vi "LVFunction_Imop_Compute_ModalWavefront.vi"(0 "HasoData":refnum<class "HasoData.lvclass">, 5 "ComputePhaseSet":refnum<class "ComputePhaseSet.lvclass">, 7 "Phase":refnum<class "Phase.lvclass">, 9 "ModalCoef.lvclass":refnum<class "ModalCoef.lvclass">, 11 "error constant":errorcluster) -> (4 "HasoData (dup)":refnum<class "HasoData.lvclass">, 6 "ComputePhaseSet (dup)":refnum<class "ComputePhaseSet.lvclass">, 8 "Phase.lvclass":refnum<class "Phase.lvclass">, 10 "ModalCoef.lvclass (dup)":refnum<class "ModalCoef.lvclass">, 15 "error out":errorcluster)   [LabVIEW 2018]
doc: "Compute phase from processed slopes of the input HasoData via modal\ncoefficients in a given basis of polynomials provided by ComputePhaseSet.\n\n<B>ComputePhaseSetIn</B> : ComputePhaseSet object.\n<B>ComputePhaseSetOut</B> : ComputePhaseSet object.\n<B>HasoData</B> : HasoData object.\n<B>ModalCoeffs</B> : ModalCoef object. Preferences are used as input, coefficients values are updated by the processing.\n<B>Phase</B> : phase object. Phase values and steps are expressed in um."
uses:
  Classes/HasoData/HasoData.lvclass
  Classes/ComputePhaseSet/ComputePhaseSet.lvclass
  Classes/Phase/Phase.lvclass
  Classes/ModalCoef/ModalCoef.lvclass
  Classes/ModalCoef/LVClass_ModalCoef Read ModalCoef.vi
  Classes/Phase/LVClasse_Phase Read SurfaceFloatWithPupil.vi
  Classes/ComputePhaseSet/LVClass_ComputePhaseSet Read ComputePhaseSet.vi
  Classes/HasoData/LVClass_HasoData Read HasoData - property.vi
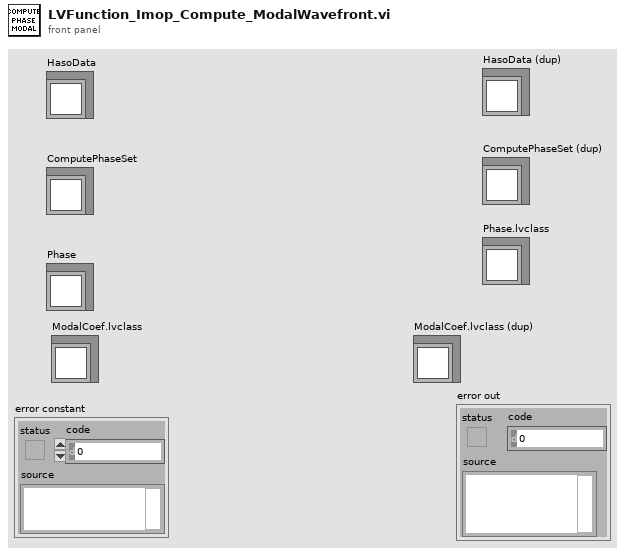
[diagram p1: front panel]
types:
  T1 = typedef "ClassID.ctl" = i64
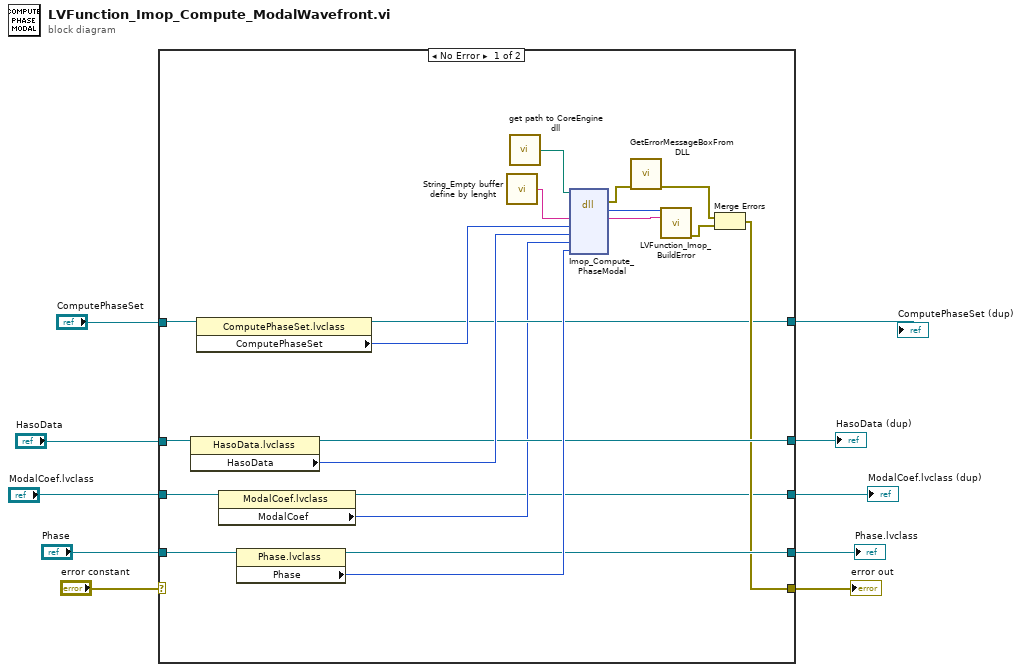
[diagram p0: block diagram]
diagram:
  n1 = case shown="No Error" "error constant" {
    selector: "error constant" -> [_ w35]
    tunnel: "HasoData" -> [w25 w34]
    tunnel: "ComputePhaseSet" -> [w24 w32]
    tunnel: [w15 w35] -> w9
    tunnel: "Phase" -> [w23 w33]
    tunnel: [w19 w33] -> w4
    tunnel: [w18 w34] -> w7
    tunnel: [w14 w32] -> w3
    tunnel: "ModalCoef.lvclass" -> [w12 w31]
    tunnel: [w11 w31] -> w1
    frame No Error {
      n2 = property class="HasoData.lvclass"(reference=w25) -> (reference out=w18:refnum<class "HasoData.lvclass">, "HasoData"=w22:T1)  [unwired: 1 in, 1 out]
      n3 = property class="ComputePhaseSet.lvclass"(reference=w24) -> (reference out=w14:refnum<class "ComputePhaseSet.lvclass">, "ComputePhaseSet"=w21:T1)  [unwired: 1 in, 1 out]
      n4 = property class="ModalCoef.lvclass"(reference=w12) -> (reference out=w11:refnum<class "ModalCoef.lvclass">, "ModalCoef"=w13:T1)  [unwired: 1 in, 1 out]
      n5 = property class="Phase.lvclass"(reference=w23) -> (reference out=w19:refnum<class "Phase.lvclass">, "Phase"=w20:T1)  [unwired: 1 in, 1 out]
      n6 = call "String_Empty buffer define by lenght.vi"() -> ("Empty buffer"=w28:string)  [unwired: 1 in]
      n7 = call "get path to CoreEngine dll.vi"() -> ("path to wavekit library"=w27:path)  [unwired: 14 in, 1 out]
      n8 = dll-call lib="D:/FLE/0.Code/CoreEngine4_Suite/LV2011_interface/DLLs/c_interface_vc100.dll" fn="Imop_Compute_PhaseModal"(path in=w27, "message"=w28, "ComputePhaseSet"=w21, "HasoData"=w22, "ModalCoeffs"=w13, "phase"=w20) -> (error out=w26:errorcluster, "return type"=w30:i32, "message"=w29:string)  [unwired: 6 in, 1 out]
      n9 = call "GetErrorMessageBoxFromDLL.vi"("error IN"=w26) -> ("error OUT"=w17:errorcluster)  [unwired: 10 in]
      n10 = call "LVFunction_Imop_BuildError.vi"("code"=w30, "String to Prepend to source (\"\")"=w29) -> ("error out"=w16:errorcluster)  [unwired: 13 in]
      n11 = Merge Errors(w17, w16) -> (w15:errorcluster)
    }
    frame Error {
    }
  }
  "error out" <- w9
  "HasoData (dup)" <- w7
  "Phase.lvclass" <- w4
  "ComputePhaseSet (dup)" <- w3
  "ModalCoef.lvclass (dup)" <- w1
